vi "Read Analogue.vi"(8 "error in (no error)":errorcluster, 11 "NI DMM4072 in":refnum<class "NI DMM4072.lvclass">) -> (0 "error out":errorcluster, 2 "Measurement":dbl format="%.5f", 3 "NI DMM4072 out":refnum<class "NI DMM4072.lvclass">)   [LabVIEW 2021, in "Concrete.lvlib" / "NI DMM4072.lvclass"]
uses:
  NI DMM4072.lvclass
  NI DMM4072.lvclass/NI DMM4072.ctl
  Harware Abstraction/MultiIO/MultiFunction IO.lvclass
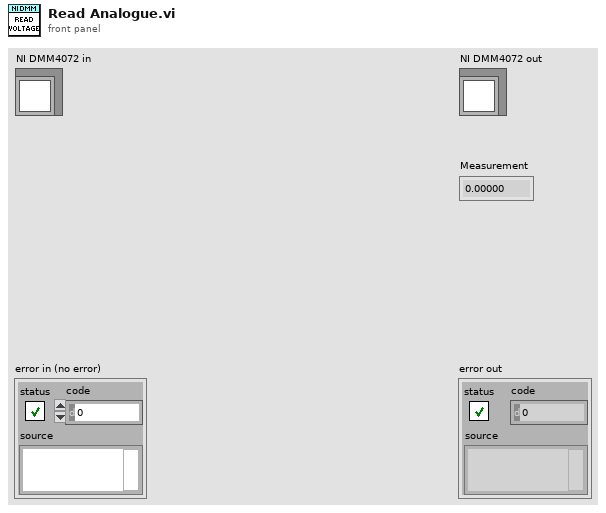
[diagram p1: front panel]
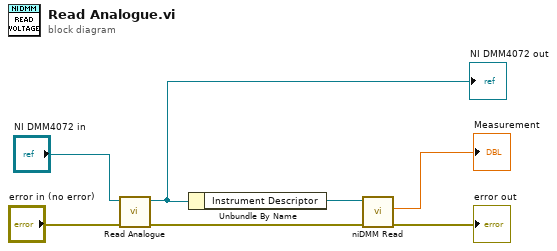
[diagram p0: block diagram]
diagram:
  n1 = call-parent "Read Analogue.vi"("error in (no error)"="error in (no error)", "DMM in"="NI DMM4072 in") -> ("error out"=w2:errorcluster, "DMM out"=w1:refnum<class "NI DMM4072.lvclass">)  [unwired: 7 in, 1 out]
  "NI DMM4072 out" <- w1
  n2 = Unbundle By Name(w1) -> ("Instrument Descriptor"=w7:refnum<k15>)
  n3 = call <instrlib>:"niDMM Read.vi"("error in (no error)"=w2, "instrument handle"=w7) -> ("error out"=→"error out":errorcluster, "Measurement"=→"Measurement":dbl)  [unwired: 1 in, 7 out]
